vi "Formula_Node_Ejercicio.vi"() -> ()   [LabVIEW 2020]
panel:
  out "Gráfico de un círculo":cluster{dbl[], dbl[]}(graph)
  out "Waveform Graph":dbl[](graph)
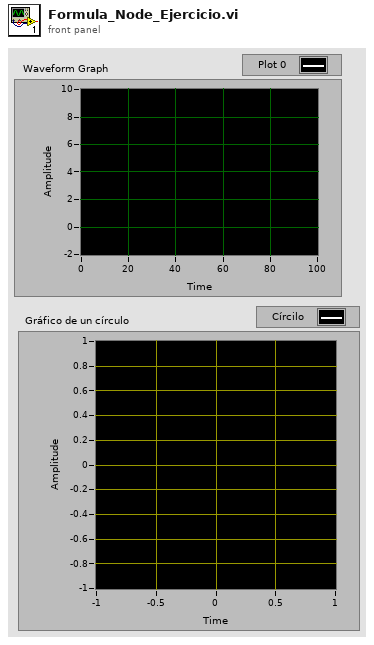
[diagram p1: front panel]
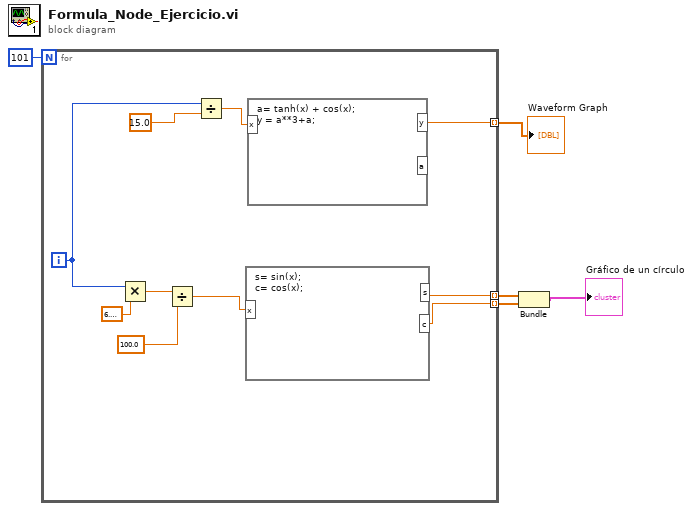
[diagram p0: block diagram]
diagram:
  n1 = for {
    N: 101 -> [_]
    tunnel: [w13] -> w4 mode=indexing
    tunnel: [w7] -> w3 mode=indexing
    tunnel: [w6] -> w2 mode=indexing
    i -> [w11]
    n2 = Multiply(x=w11, y=6.283185307179586) -> (x*y=w10:dbl)
    n3 = Divide(x=w10, y=100.0) -> (x/y=w8:dbl)
    n4 = Divide(x=w11, y=15.0) -> (x/y=w14:dbl)
    n5 = formula code="s= sin(x);\nc= cos(x);"("x"=w8) -> ("s"=w7:dbl, "c"=w6:dbl)
    n6 = formula code="a= tanh(x) + cos(x);\ny = a**3+a;"("x"=w14) -> ("y"=w13:dbl)  [unwired: 1 out]
  }
  "Waveform Graph" <- w4
  n7 = Bundle(w3, w2) -> (→"Gráfico de un círculo":cluster{dbl[], dbl[]})  [unwired: 1 in]
